vi "Available Commands.vi"() -> ()   [LabVIEW 2025]
panel:
  in  "Command Type":enum16{"Set", "Get"}(ring)
  in  "Command":T1(ring)
  in  "Unit":string
  in  "Value":i32=2
  in  "byte count":u32
  out "Read Buffer":string
  in  "Bytes to Read":u32=52
  out "Serial Number":string
  out "Device":string
  out "Connected?":bool
  in  "Port":string="3000"
  in  "IP Address":string="192.168.1.99"
  in  "Error In":errorcluster
  out "Error Out":errorcluster
  out "Command":string
  in  "Channel":i32
  out "Query Only":bool[](array[boolean])
  out "Commands":string[](array[string])
  out "No Query Form":bool[](array[boolean])
  out "Cleaned":string[](array[string])
  in  "String":string="AFGControl:CSCopy (No Query Form).......................................................................................3\n*CLS (No Query Form)...............................................................................................................3\nCOUNter:COUPing.....................................................................................................................3\nCOUNter:DUTYcycle? (Query Only)...........................................................................................4\nCOUNter:FREQ? (Query Only)...................................................................................................4\nCOUNter:HFR ............................................................................................................................5\nCOUNter:PERiod? (Query Only) ................................................................................................5\nCOUNter:PULSewidth? (Query Only) ........................................................................................6\nCOUNter:SENSitivity..................................................................................................................6\nCOUNter:TRIGger......................................................................................................................7\nDISPlay:BRIGhtness...................................................................................................................7\nDISPlay:SAVer:DELay .................................................................................................................8\nDISPlay:SAVer:IMMediate (No Query Form) .............................................................................8\nDISPlay:SAVer[:STATe]................................................................................................................9\nHCOPy:SDUMp:DATA? (Query Only) .........................................................................................9\nHCOPy:SDUMp[:IMMediate] (No Query Form).......................................................................10\n*IDN? (Query Only).................................................................................................................10\nMMEMory:CATalog? (Query Only)..........................................................................................11\nMMEMory:CDIRectory ............................................................................................................11\nMMEMory:DELete (No Query Form) ......................................................................................12\nOUTPut[1|2]:IMPedance ........................................................................................................12\nOUTPut[1|2][:STATe]...............................................................................................................13\n*RCL (No Query Form) ............................................................................................................13\n*RST (No Query Form) ............................................................................................................14\n*SAV (No Query Form) ............................................................................................................14\n[SOURce[1|2]]:AM[:DEPTh] ....................................................................................................15\n[SOURce[1|2]]:AM:INTernal:FREQuency ................................................................................15\n[SOURce[1|2]]:AM:INTernal:FUNCtion ...................................................................................16\n[SOURce[1|2]]:AM:INTernal:FUNCtion:EFILe..........................................................................16\n[SOURce[1|2]]:AM:SOURce ....................................................................................................17\n[SOURce[1|2]]:AM:STATe ........................................................................................................17\n[SOURce[1|2]]:ASKey[:AMPLitude].........................................................................................18\n[SOURce[1|2]]:ASKey:INTernal:RATE ......................................................................................19\n[SOURce[1|2]]:ASKey:SOURce ................................................................................................19\n[SOURce[1|2]]:ASKey:STATe....................................................................................................20\n[SOURce[1|2]]:BPSKey:DATA...................................................................................................20\n[SOURce[1|2]]:BPSKey:INTernal:RATE ....................................................................................21\n[SOURce[1|2]]:BPSKey:PHASe ................................................................................................21\n[SOURce[1|2]]:BPSKey:STATe..................................................................................................22\n[SOURce[1|2]]:BURSt:GATE:POLarity......................................................................................22\n[SOURce[1|2]]:BURSt:INTernal:PERiod ...................................................................................23\n[SOURce[1|2]]:BURSt:MODE ..................................................................................................23\n[SOURce[1|2]]:BURSt:NCYCles................................................................................................24\n[SOURce[1|2]]:BURSt:SOURce................................................................................................25\n[SOURce[1|2]]:BURSt:STATe....................................................................................................25\n[SOURce[1|2]]:FM[:DEViation]...............................................................................................26\n[SOURce[1|2]]:FM:INTernal:FREQuency.................................................................................26\n[SOURce[1|2]]:FM:INTernal:FUNCtion....................................................................................27\n[SOURce[1|2]]:FM:INTernal:FUNCtion:EFILe ..........................................................................27\n[SOURce[1|2]]:FM:SOURce.....................................................................................................28\n[SOURce[1|2]]:FM:STATe.........................................................................................................28\n[SOURce[1|2]]:FREQuency:CENTer.........................................................................................29\n[SOURce[1|2]]:FREQuency:CONCurrent.................................................................................30\n[SOURce[1|2]]:FREQuency[:FIXed] .........................................................................................30\n[SOURce[1|2]]:FREQuency:SPAN............................................................................................31\n[SOURce[1|2]]:FREQuency:STARt ...........................................................................................31\n[SOURce[1|2]]:FREQuency:STOP ............................................................................................32\n[SOURce[1|2]]:FSKey[:FREQuency].........................................................................................33\n[SOURce[1|2]]:FSKey:INTernal:RATE.......................................................................................33\n[SOURce[1|2]]:FSKey:SOURce.................................................................................................34\n[SOURce[1|2]]:FSKey:STATe ....................................................................................................34\n[SOURce[1|2]]:3FSKey[:FREQuency].......................................................................................35\n[SOURce[1|2]]:3FSKey:INTernal:RATE.....................................................................................35\n[SOURce[1|2]]:3FSKey:STATe ..................................................................................................36\n[SOURce[1|2]]:4FSKey[:FREQuency].......................................................................................36\n[SOURce[1|2]]:4FSKey:INTernal:RATE.....................................................................................37\n[SOURce[1|2]]:4FSKey:STATe ..................................................................................................38\n[SOURce[1|2]]:FUNCtion:EFILe...............................................................................................38\n[SOURce[1|2]]:FUNCtion:RAMP:SYMMetry ...........................................................................39\n[SOURce[1|2]]:FUNCtion[:SHAPe] ..........................................................................................39\n[SOURce[1|2]]:HARMonic:AMPL ............................................................................................41\n[SOURce[1|2]]:HARMonic:ORDEr...........................................................................................41\n[SOURce[1|2]]:HARMonic:PHASe ...........................................................................................42\n[SOURce[1|2]]:HARMonic:TYPe..............................................................................................42\n[SOURce[1|2]]:MOD:STATe .....................................................................................................43\n[SOURce[1|2]]:OSKey:INTernal:RATE ......................................................................................43\n[SOURce[1|2]]:OSKey:STATe....................................................................................................44\n[SOURce[1|2]]:OSKey:TIME ....................................................................................................45\n[SOURce[1|2]]:PHASe[:ADJust]...............................................................................................45\n[SOURce[1|2]]:PHASe:INITiate (No Query Form) ...................................................................46\n[SOURce[1|2]]:PM[:DEViation]...............................................................................................46\n[SOURce[1|2]]:PM:INTernal:FREQuency.................................................................................47\n[SOURce[1|2]]:PM:INTernal:FUNCtion ...................................................................................47\n[SOURce[1|2]]:PM:INTernal:FUNCtion:EFILe..........................................................................48\n[SOURce[1|2]]:PM:SOURce ....................................................................................................49\n[SOURce[1|2]]:PM:STATe ........................................................................................................49\n[SOURce[1|2]]:PSKey[:DEViation]...........................................................................................50\n[SOURce[1|2]]:PSKey:INTernal:RATE.......................................................................................50\n[SOURce[1|2]]:PSKey:SOURce ................................................................................................51\n[SOURce[1|2]]:PSKey:STATe ....................................................................................................51\n[SOURce[1|2]]:PULSe:DCYCle .................................................................................................52\n[SOURce[1|2]]:PULSe:TRANsition[:LEADing]..........................................................................52\n[SOURce[1|2]]:PULSe:TRANsition:TRAiling.............................................................................53\n[SOURce[1|2]]:PULSe:WIDTh..................................................................................................53\n[SOURce[1|2]]:PWM:INTernal:FREQuency .............................................................................54\n[SOURce[1|2]]:PWM:INTernal:FUNCtion................................................................................55\n[SOURce[1|2]]:PWM:INTernal:FUNCtion:EFILe ......................................................................55\n[SOURce[1|2]]:PWM:SOURce.................................................................................................56\n[SOURce[1|2]]:PWM:STATe.....................................................................................................56\n[SOURce[1|2]]:PWM[:DEViation]:DCYCle...............................................................................57\n[SOURce[1|2]]:SWEep:SOURce...............................................................................................57\n[SOURce[1|2]]:SWEep:SPACing...............................................................................................58\n[SOURce[1|2]]:SWEep:STATe ..................................................................................................58\n[SOURce[1|2]]:SWEep:TIME ...................................................................................................59\n[SOURce[1|2]]:VOLTage[:LEVel][:IMMediate]:OFFSet ............................................................60\n[SOURce[1|2]]:VOLTage[:LEVel][:IMMediate][:AMPLitude] ...................................................60\nSYSTem:BEEPer[:IMMediate] (No Query Form) ......................................................................61\nSYSTem:BEEPer:STATe..............................................................................................................61\nSYSTem:ERRor[:NEXT]? (Query Only) ......................................................................................62\nSYSTem:KLOCk[:STATe].............................................................................................................62\nSYSTem:LANguage...................................................................................................................63\nSYSTem:POWeron....................................................................................................................63\nSYSTem:RESTART .....................................................................................................................64\nSYSTem:VERSion? (Query Only)...............................................................................................64\nTRACe|DATA:CATalog? (Query Only).......................................................................................65\nTRACe|DATA:COPY (No Query Form)......................................................................................65\nTRACe|DATA[:DATA]................................................................................................................66\nTRACe|DATA[:DATA]:VALue.....................................................................................................66\nTRACe|DATA:POINts................................................................................................................67\n*TRG (No Query Form)............................................................................................................67"
  # "http://www.farnell.com/datasheets/3668638.pdf"
  # "https://www.farnell.com/datasheets/3200197.pdf?_gl=1*1d7nxhe*_gcl_aw*R0NMLjE3NTAwNzg3NjIuQ2p3S0NBandnYl9DQmhCTUVpd0EwcDNvT0daeU5GNjJyQjM4MEVMU1pTVWtkNWFfbDUzOFVlaDZrTDhmcGgzaFdPQW9HRF9RVDFCS1BSb0NZRmdRQXZEX0J3RQ..*_gcl_au*MjE0MzIzMTA5MC4xNzQ5NTg3ODM3"
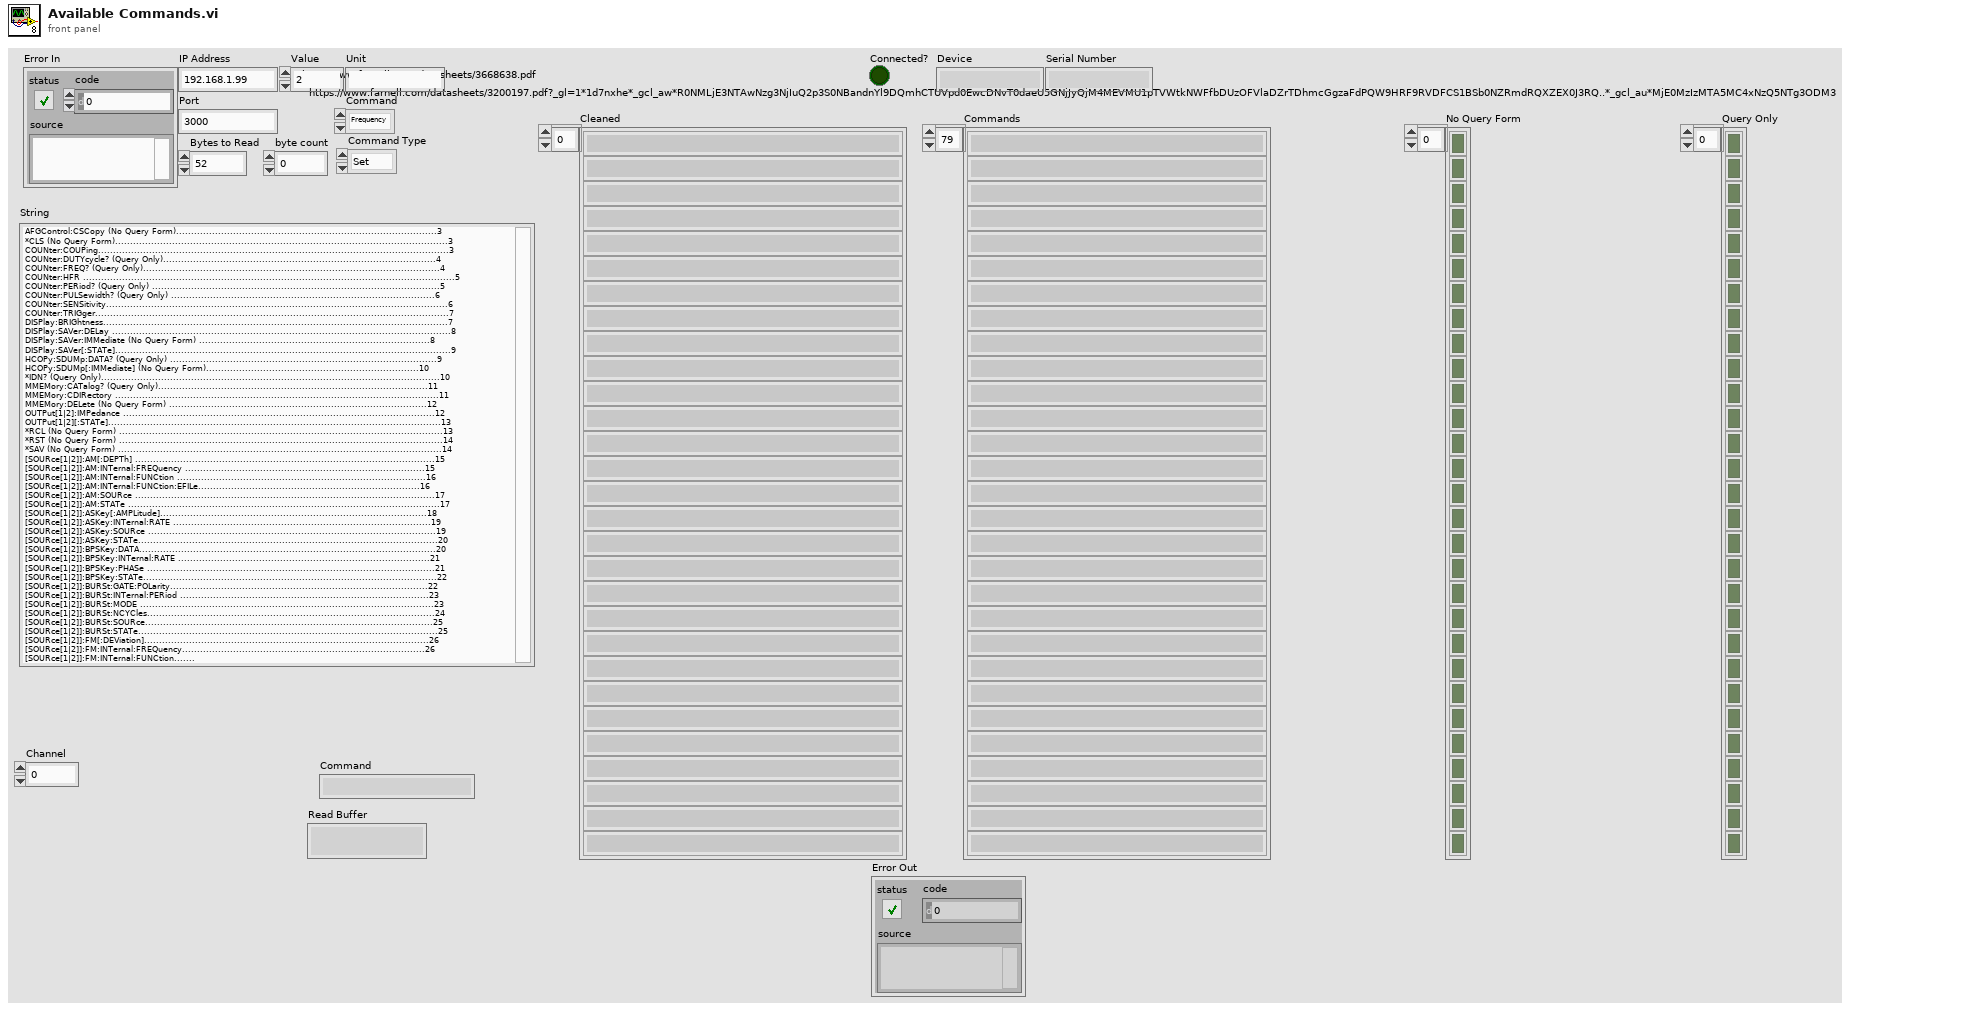
[diagram p1: front panel]
types:
  T1 = enum16{"Frequency", "Voltage Level", "Voltage Offset", "Phase", "Phase Sync", "Wave Type"}
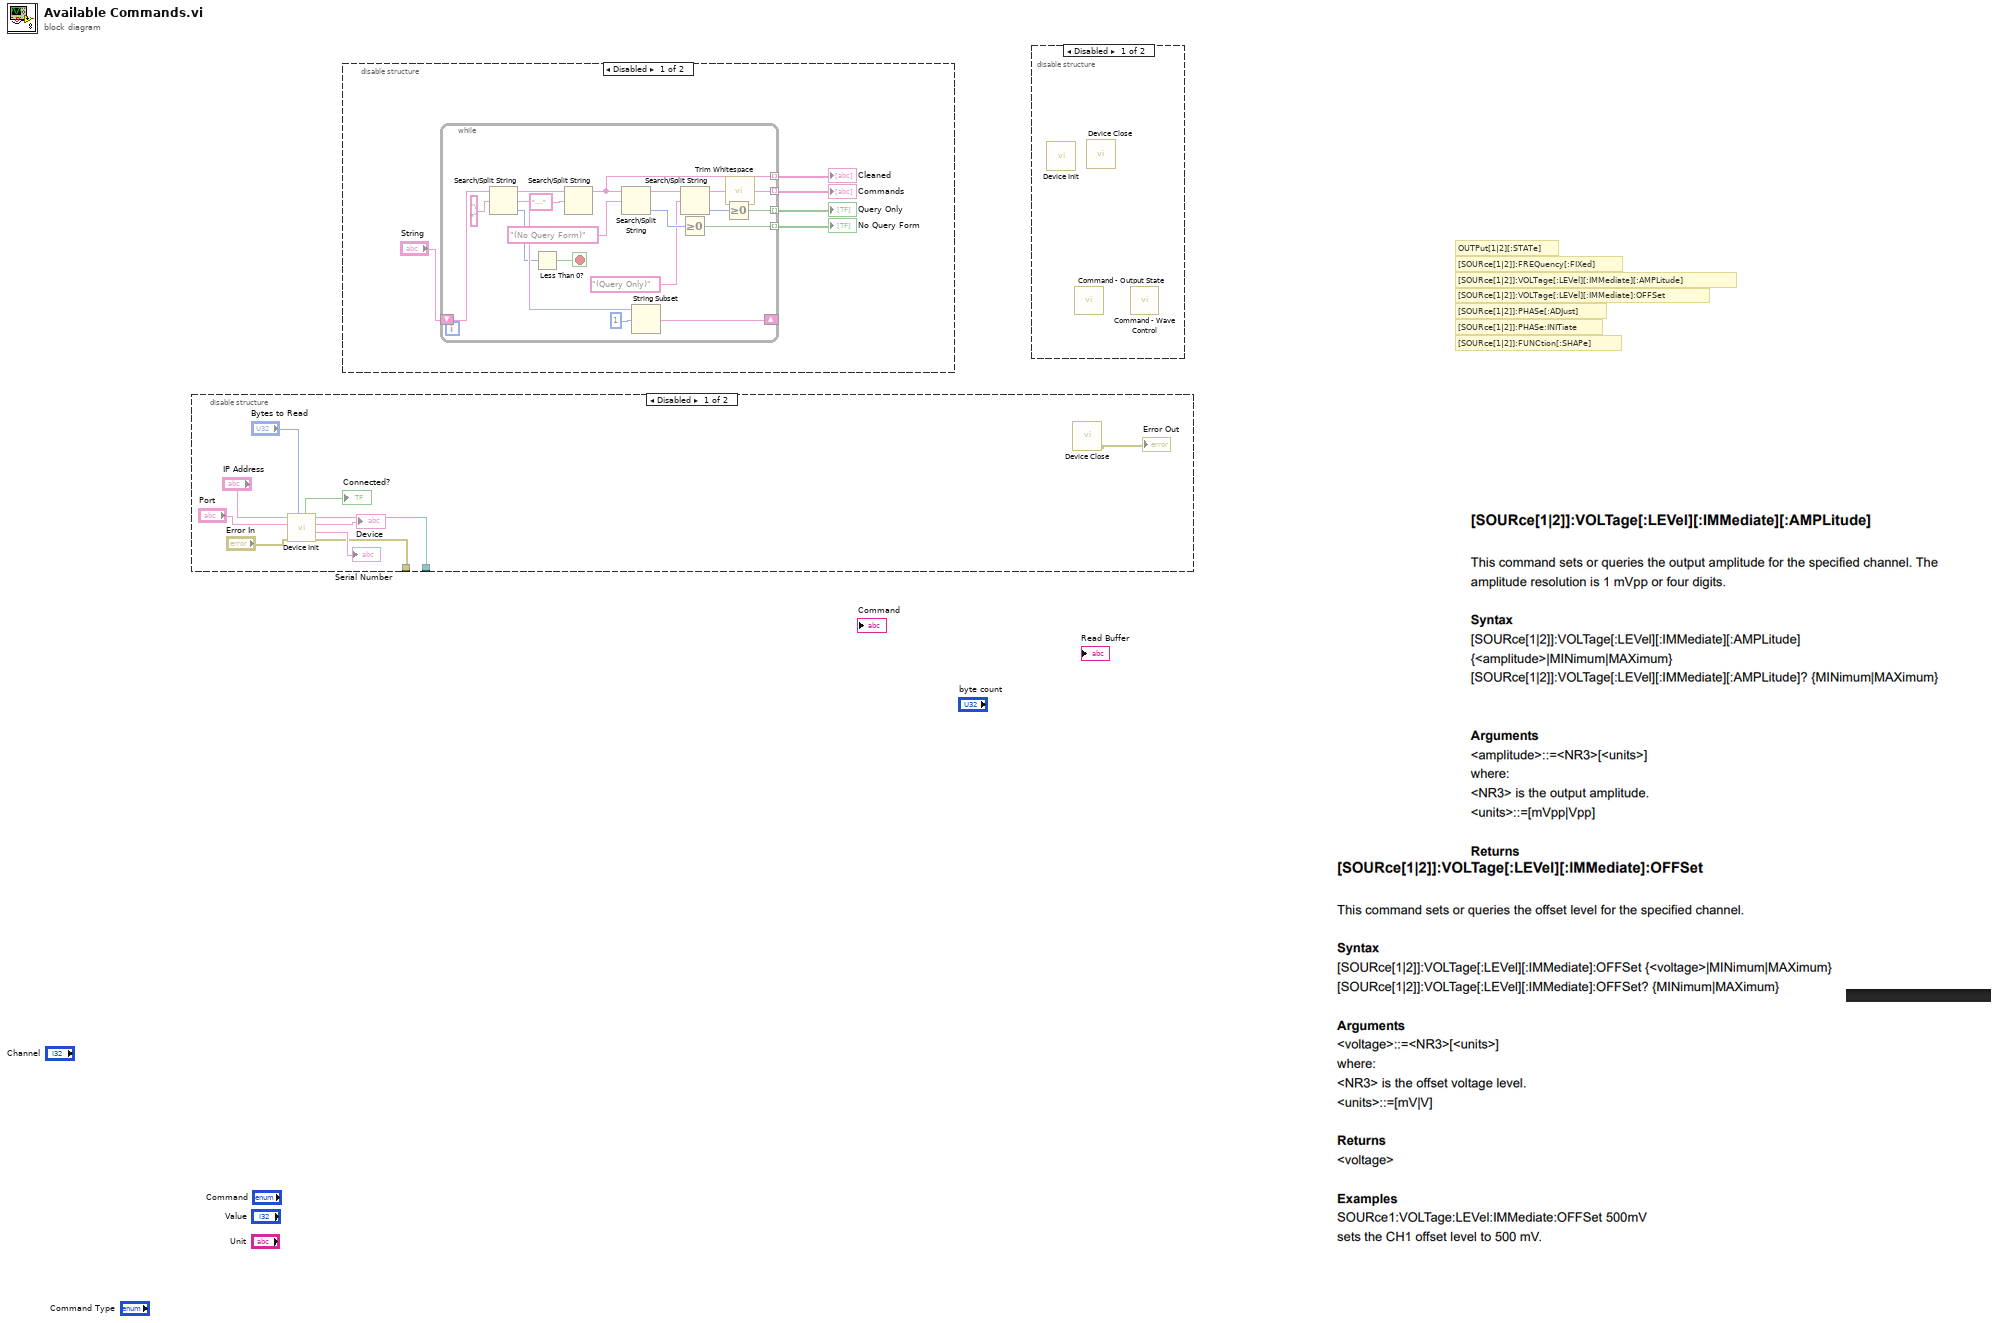
[diagram p0: block diagram]
diagram:
  # "[SOURce[1|2]]:FUNCtion[:SHAPe]"
  # "[SOURce[1|2]]:PHASe:INITiate"
  # "[SOURce[1|2]]:PHASe[:ADJust]"
  # "[SOURce[1|2]]:VOLTage[:LEVel][:IMMediate]:OFFSet"
  # "[SOURce[1|2]]:VOLTage[:LEVel][:IMMediate][:AMPLitude]"
  # "OUTPut[1|2][:STATe]"
  # "[SOURce[1|2]]:FREQuency[:FIXed]"
  n1 = disable-structure shown="Disabled" {
    disable-tunnel: [w10 _] -> _
    disable-tunnel: [w1 _] -> _
    frame Disabled {
      n2 = call "Device Init.vi"("Bytes to Read"="Bytes to Read", "Error In"="Error In", "Port"="Port", "IP Address"="IP Address") -> ("Error Out"=w1:errorcluster, "Serial Number"=→"Serial Number":string, "Device"=→"Device":string, "VISA resource name"=w10:refnum<visa-resource-name>, "Connected?"=→"Connected?":bool)  [unwired: 3 in]
      n3 = call "Device Close.vi"() -> ("Error Out"=→"Error Out":errorcluster)  [unwired: 11 in]
    }
    frame Enabled {
    }
  }
  n4 = disable-structure shown="Disabled" {
    frame Disabled {
      n5 = while {
        shift-right: [w33] -> _
        shift-left: "String" -> [w34]
        tunnel: [w25] -> w13 mode=indexing
        tunnel: [w22] -> w14 mode=indexing
        tunnel: [w17] -> w12 mode=indexing
        tunnel: [w18] -> w11 mode=indexing
        stop <- w29 stop-if-true
        n6 = Search/Split String(string=w34, search string/char (-)="\n") -> (substring before match=w24:string, match + rest of string=w31:string, offset of match=w30:i32)  [unwired: 1 in]
        n7 = Less Than 0?(x=w30) -> (x < 0?=w29:bool)
        n8 = Search/Split String(string=w24, search string/char (-)="....") -> (substring before match=w22:string)  [unwired: 1 in, 2 out]
        n9 = Search/Split String(string=w22, search string/char (-)="(No Query Form)") -> (substring before match=w21:string, offset of match=w26:i32)  [unwired: 1 in, 1 out]
        n10 = String Subset(string=w31, offset (0)=1) -> (substring=w33:string)  [unwired: 1 in]
        n11 = Greater Or Equal To 0?(x=w26) -> (x >= 0?=w25:bool)
        n12 = Search/Split String(string=w21, search string/char (-)="(Query Only)") -> (substring before match=w16:string, offset of match=w19:i32)  [unwired: 1 in, 1 out]
        n13 = Greater Or Equal To 0?(x=w19) -> (x >= 0?=w18:bool)
        n14 = call <vilib>:"Trim Whitespace.vi"("string"=w16) -> ("trimmed string"=w17:string)  [unwired: 1 in]
      }
      "Cleaned" <- w14
      "No Query Form" <- w13
      "Commands" <- w12
      "Query Only" <- w11
    }
    frame Disabled {
    }
  }
  n15 = disable-structure shown="Disabled" {
    frame Disabled {
      n16 = call "Device Init.vi"() -> ()  [unwired: 7 in, 5 out]
      n17 = call "Command - Output State.vi"() -> ()  [unwired: 9 in, 3 out]
      n18 = call "Device Close.vi"() -> ()  [unwired: 11 in, 1 out]
      n19 = call "Command - Wave Control.vi"() -> ()  [unwired: 13 in, 3 out]
    }
    frame Enabled {
    }
  }
